vi "StepNameLengthRuleConstants.vi"() -> ()   [LabVIEW 2011]
panel:
  in  "Default Maximum Step Name Length":i32=15
  in  "Maximum Step Name Length Property Name":string="MaximumStepNameLength"
  in  "CheckStepNameLength Rule Id":string="NI_CheckStepNameLengthLVExample"
  # "Constants used by the CheckStepNameLength rule module.\nThe Rule Id constant must match the Rule Id specified in the\nEdit Rule dialog box."
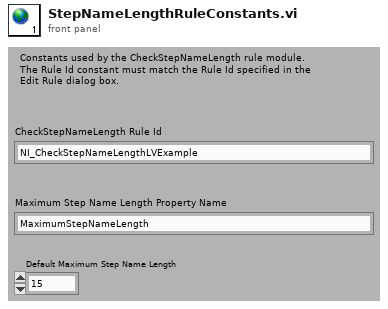
[diagram p1: front panel]
diagram:
